vi "Add Channel.vi"(8 "error in":errorcluster, 10 "hardwareChannel":i32, 11 "parameter file in":refnum<k24>) -> (0 "error out":errorcluster, 2 "new channel":refnum<k24>, 3 "parameter file out":refnum<k24>)   [LabVIEW 2020, in "Ballard_1553_Parameter_ni.lvlib"]
uses:
  Ballard_1553_Parameter_ni.lvlib
  C:/Users/Administrator/Desktop/GIT/Ballard-Arinc-429-XML-Generator/Source/Assemblies/Ballard_1553_Parameter_ni/bin/Debug/Ballard_1553_Parameter_ni.dll
  Assemblies/Ballard_1553_Parameter_ni/bin/Debug/Ballard_1553_Parameter_ni.dll
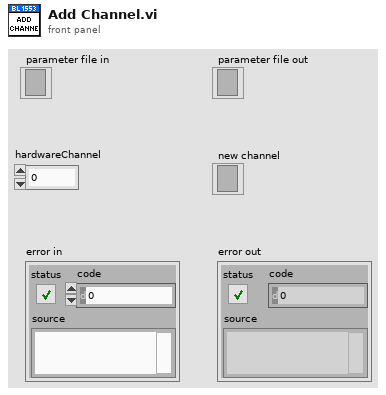
[diagram p1: front panel]
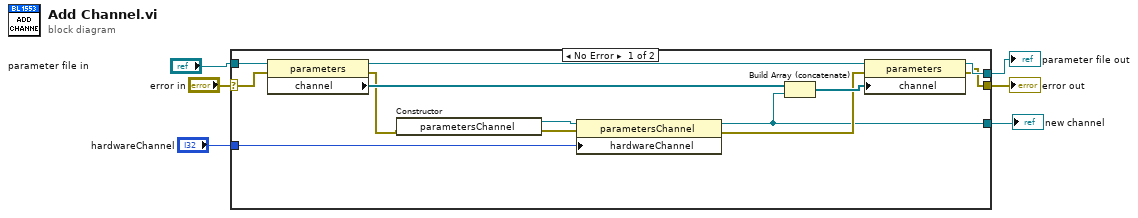
[diagram p0: block diagram]
diagram:
  n1 = case shown="No Error" "error in" {
    selector: "error in" -> [w18 w20]
    tunnel: [w15 w21] -> w6
    tunnel: [w14 w20] -> w5
    tunnel: "parameter file in" -> [w19 w21]
    tunnel: [w10 _] -> w1
    tunnel: "hardwareChannel" -> [w11 _]
    frame No Error {
      n2 = property class="parameters"(reference=w19, error in=w18) -> (reference out=w16:refnum<k24>, error out=w9:errorcluster, "channel"=w17:refnum<k24>[])
      n3 = constructor class="parametersChannel"(error in=w9) -> (reference out=w7:refnum<k24>, error out=w8:errorcluster)  [unwired: 2 in, 1 out]
      n4 = property class="parametersChannel"(reference=w7, error in=w8, "hardwareChannel"=w11) -> (reference out=w10:refnum<k24>, error out=w12:errorcluster)
      n5 = Build Array (concatenate)(w17, w10) -> (w13:refnum<k24>[])
      n6 = property class="parameters"(reference=w16, error in=w12, "channel"=w13) -> (reference out=w15:refnum<k24>, error out=w14:errorcluster)
    }
    frame Error {
    }
  }
  "parameter file out" <- w6
  "error out" <- w5
  "new channel" <- w1
